vi "PQsyncQueryCommand.vi"(8 "error in (no error)":errorcluster, 9 "query":string, 11 "conn":u32) -> (0 "error out":errorcluster, 1 "PQresultStatus":T1(ring), 2 "PGresult":u32, 3 "conn out":u32, 4 "PQresultErrorMessage":string)   [LabVIEW 2019, in "libpqutility.lvlib"]
doc: "Synchrounus Communication with PostgreSQL Database.\nSee PostgreSQL c-lib doku for further information."
uses:
  libpqutility.lvlib
  libpqlv/libpqlv.lvlib
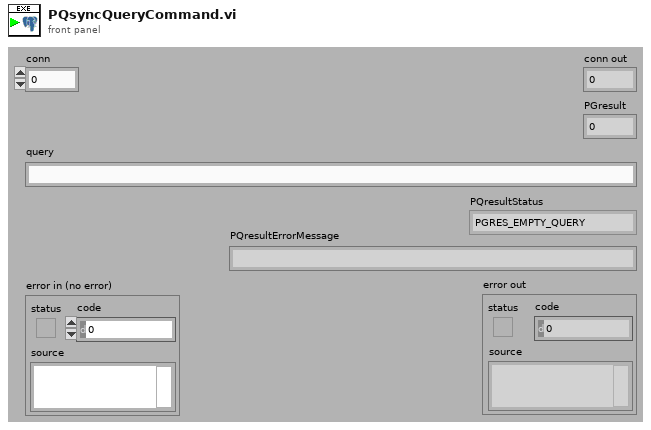
[diagram p1: front panel]
types:
  T1 = enum32{"PGRES_EMPTY_QUERY", "PGRES_COMMAND_OK", "PGRES_TUPLES_OK", "PGRES_COPY_OUT", "PGRES_COPY_IN", "PGRES_BAD_RESPONSE", "PGRES_NONFATAL_ERROR", "PGRES_FATAL_ERROR"}
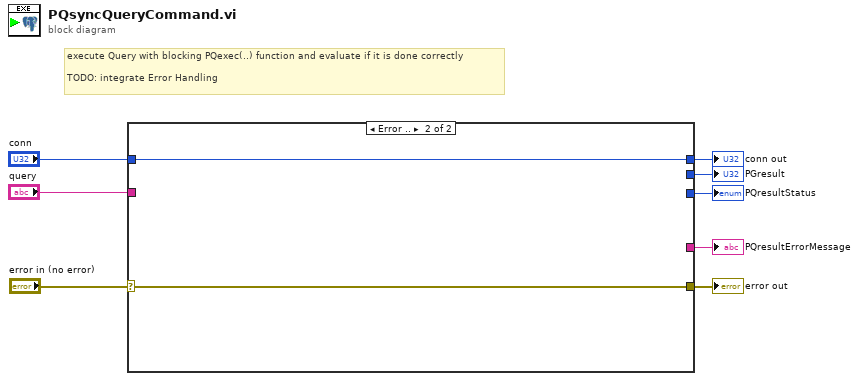
[diagram p0: block diagram]
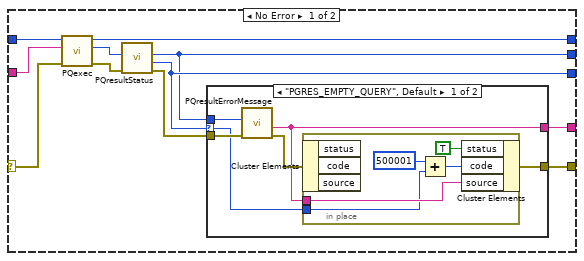
[diagram p2: hidden frame]
diagram:
  # "execute Query with blocking PQexec(..) function and evaluate if it is done correctly\n\nTODO: integrate Error Handling"
  n1 = case shown="Error .." "error in (no error)" {
    selector: "error in (no error)" -> [w10 w32]
    tunnel: "query" -> [w9 _]
    tunnel: "conn" -> [w18 w33]
    tunnel: [w15 w32] -> w6
    tunnel: [w14 _] -> w5
    tunnel: [w13 _] -> w4
    tunnel: [w12 w33] -> w3
    tunnel: [w11 _] -> w2
    frame No Error {
      n2 = call "PQexec.vi"("error in (no error)"=w10, "query"=w9, "conn"=w18) -> ("error out"=w17:errorcluster, "PGresult"=w19:u32, "conn out"=w12:u32)  [unwired: 6 in]
      n3 = call "PQresultStatus.vi"("error in (no error)"=w17, "res"=w19) -> ("error out"=w16:errorcluster, "PQresultStatus"=w14:T1, "res out"=w11:u32)  [unwired: 7 in]
      n4 = case shown="\"PGRES_EMPTY_QUERY\", Default" w14 {
        selector: w14 -> [w21 _]
        tunnel: w16 -> [w24 w31]
        tunnel: [w20 w31] -> w15
        tunnel: w11 -> [w25 _]
        tunnel: [w22 _] -> w13
        frame "PGRES_EMPTY_QUERY", Default {
          n5 = call "PQresultErrorMessage.vi"("error in (no error)"=w24, "res"=w25) -> ("error out"=w23:errorcluster, "PQresultErrorMessage"=w22:string)  [unwired: 7 in, 1 out]
          n6 = in-place {
            in-place-border: w22 -> [w30]
            in-place-border: w21 -> [w27]
            n7 = in-place-cluster #1(w23) -> ()  [unwired: 3 out]
            n8 = Add(x=u32 500001, y=w27) -> (x+y=w26:u32)
            n9 = in-place-cluster #1("status"=TRUE, "code"=w26, "source"=w30) -> (w20:errorcluster)
          }
        }
        frame "PGRES_COMMAND_OK" {
        }
      }
    }
    frame Error {
    }
  }
  "PQresultStatus" <- w5
  "PQresultErrorMessage" <- w4
  "PGresult" <- w2
  "conn out" <- w3
  "error out" <- w6
